vi "Init.vi"(9 "Project:Active Project":refnum<vi>, 10 "NI.LV.Dialog Instance":refnum<vi>) -> (0 "error out":errorcluster, 3 "_Rescript Msg out":refnum<class "_Msg Rescript.lvclass">)   [LabVIEW 2021, in "_Msg Rescript.lvlib" / "_Msg Rescript.lvclass"]
uses:
  _Msg Rescript.lvclass
  _Msg Rescript.lvclass/_Msg Rescript.ctl
  <vilib>/Utility/EditLVProj/Edit LVProj.lvlib
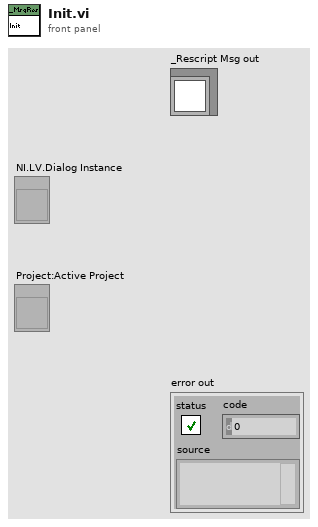
[diagram p1: front panel]
types:
  T1 = typedef "Edit LVProj.lvlib/Library And VI References.ctl" = cluster{"Target Reference":refnum<vi>, "VI References":refnum<vi>[], "Library References":refnum<vi>[]}
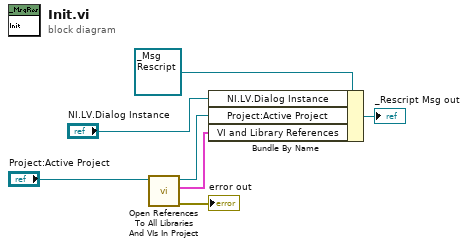
[diagram p0: block diagram]
diagram:
  n1 = call <vilib>:"Open References To All Libraries And VIs In Project.vi"("Project in"="Project:Active Project") -> ("error out"=→"error out":errorcluster, "VI and Library References"=w1:T1[], "Project out"=w3:refnum<vi>)  [unwired: 8 in]
  n2 = Bundle By Name(cluster=refnum<class "_Msg Rescript.lvclass"> refnum ("_Rescript Msg out"), "NI.LV.Dialog Instance"="NI.LV.Dialog Instance", "Project:Active Project"=w3, "VI and Library References"=w1) -> (→"_Rescript Msg out":refnum<class "_Msg Rescript.lvclass">)
